vi "Get Array of Record Data.vi"(8 "error in (no error)":errorcluster, 11 "Record in":refnum<class "Record.lvclass">) -> (0 "error out":errorcluster, 2 "Array of Record Data":variant[](array[variant]), 3 "Record out":refnum<class "Record.lvclass">)   [LabVIEW 2017, in "Error Log.lvlib" / "Record.lvclass"]
uses:
  Record.lvclass
  Record.lvclass/Record.ctl
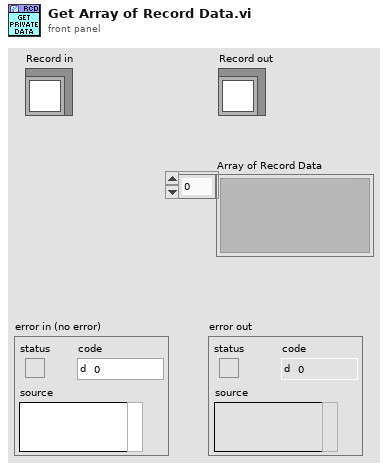
[diagram p1: front panel]
types:
  T1 = typedef "Error Log.lvlib/Record.lvclass/privateData.ctl" = cluster{"Level":string, "Time Stamp":string, "Message":string}
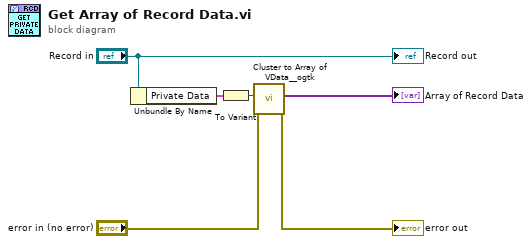
[diagram p0: block diagram]
diagram:
  n1 = Unbundle By Name("Record in") -> ("Private Data"=w4:T1)
  n2 = To Variant(anything=w4) -> (Variant=w5:variant)
  n3 = call <userlib>:"Cluster to Array of VData__ogtk.vi"("error in (no error)"="error in (no error)", "Cluster"=w5) -> ("error out"=→"error out":errorcluster, "Array of VData"=→"Array of Record Data":variant[])  [unwired: 8 in]
  "Record out" <- "Record in"
